vi "get paths in variant helper.vi"(8 "error in (no error)":errorcluster, 9 "index":i32, 10 "Parent Name":string, 11 "variant":variant) -> (0 "error out":errorcluster, 1 "structure":bool[](array[boolean]), 2 "paths":string[](array[string]))   [LabVIEW 2016, in "JSFL Variant Support.lvlib"]
uses:
  JSFL Variant Support.lvlib
  <vilib>/Utility/Data Type/NI_Data Type.lvlib
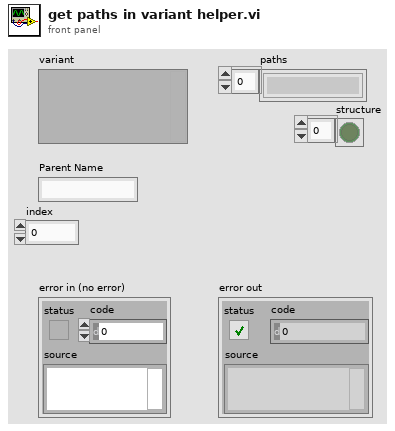
[diagram p1: front panel]
types:
  T1 = typedef "NI_Data Type.lvlib/Data Type.ctl" = enum8{"Invalid Type", "Void", "I8", "I16", "I32", "I64", "U8", "U16", "U32", "U64", "Single Float", "Double Float", "Extended Float", "Single Complex", "Double Complex", "Extended Complex", "Enum U8", "Enum U16", "Enum U32", "Enum U64", "Single Float With Unit", "Double Float With Unit", "Extended Float With Unit", "Single Complex with Unit", "Double Complex with Unit", "Extended Complex with Unit", "Boolean", "String", "Path", "Picture", "Tag", "Array", "Cluster", "Variant", "LV Variant", "Waveform", "Timestamp", "Digital Waveform", "Digital Data", "ExpressData", "Refnum", "External Data", "VI", "Poly VI", "LabVIEW Class Instance", "Fixed Point"}
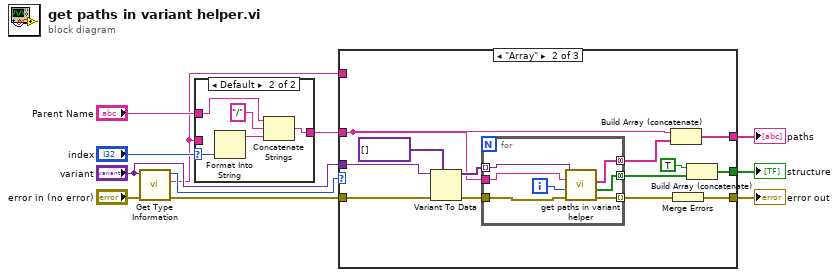
[diagram p0: block diagram]
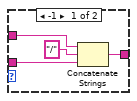
[diagram p2: hidden frame]
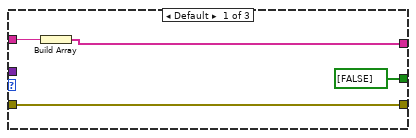
[diagram p3: hidden frame]
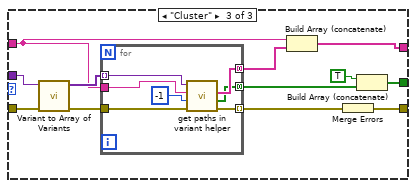
[diagram p4: hidden frame]
diagram:
  n1 = call <vilib>:"Get Type Information.vi"("error in (no error)"="error in (no error)", "Variant"="variant") -> ("error out"=w7:errorcluster, "Name"=w3:string, "Type"=w10:T1)  [unwired: 5 in, 2 out]
  n2 = case shown="Default" "index" {
    selector: "index" -> [_ w17]
    tunnel: "Parent Name" -> [w14 w19]
    tunnel: w3 -> [w13 _]
    tunnel: [w12 w18] -> w2
    frame -1 {
      n3 = Concatenate Strings(w14, "/" ("string"), w13) -> (w12:string)
    }
    frame Default {
      n4 = Format Into String(w17) -> (resulting string=w16:string)  [unwired: 3 in, 1 out]
      n5 = Concatenate Strings(w19, "/" ("string"), w16) -> (w18:string)
    }
  }
  n6 = case shown="\"Array\"" w10 {
    tunnel: "variant" -> [_ w37 w52]
    tunnel: w3 -> [_ _ _]
    tunnel: [w24 w33 w55] -> w8
    tunnel: w7 -> [w23 w32 w50]
    tunnel: [w23 w29 w53] -> w6
    tunnel: w2 -> [w22 w28 w48]
    tunnel: [bool[] [FALSE] w25 w46] -> w1
    frame Default {
      n7 = Build Array(w22) -> (w24:string[])
    }
    frame "Array" {
      n8 = Variant To Data(error in=w32, type=variant[] [], Variant=w37) -> (data=w35:variant[], error out=w31:errorcluster)
      n9 = for {
        tunnel: w35 -> [w44] mode=indexing
        tunnel: w28 -> [w43]
        tunnel: [w42] -> w34 mode=concatenating
        tunnel: w31 -> [w41]
        tunnel: [w40] -> w30 mode=indexing
        tunnel: [w38] -> w27 mode=concatenating
        i -> [w39]
        n10 = call "get paths in variant helper.vi"("error in (no error)"=w41, "index"=w39, "Parent Name"=w43, "variant"=w44) -> ("error out"=w40:errorcluster, "structure"=w38:bool[], "paths"=w42:string[])  [unwired: 5 in]
      }
      n11 = Build Array (concatenate)(w28, w34) -> (w33:string[])
      n12 = Merge Errors(w30) -> (w29:errorcluster)
      n13 = Build Array (concatenate)(TRUE ("Boolean"), w27) -> (w25:bool[])
    }
    frame "Cluster" {
      n14 = call "Variant to Array of Variants.vi"("error in (no error)"=w50, "variant"=w52) -> ("error out"=w49:errorcluster, "Array"=w51:variant[])  [unwired: 8 in]
      n15 = for {
        tunnel: w51 -> [w63] mode=indexing
        tunnel: w48 -> [w62]
        tunnel: [w61] -> w56 mode=concatenating
        tunnel: w49 -> [w60]
        tunnel: [w59] -> w54 mode=indexing
        tunnel: [w57] -> w45 mode=concatenating
        n16 = call "get paths in variant helper.vi"("error in (no error)"=w60, "index"=-1, "Parent Name"=w62, "variant"=w63) -> ("error out"=w59:errorcluster, "structure"=w57:bool[], "paths"=w61:string[])  [unwired: 5 in]
      }
      n17 = Build Array (concatenate)(w48, w56) -> (w55:string[])
      n18 = Merge Errors(w54) -> (w53:errorcluster)
      n19 = Build Array (concatenate)(TRUE, w45) -> (w46:bool[])
    }
  }
  "paths" <- w8
  "error out" <- w6
  "structure" <- w1
